vi "Multi_FTP_Put.vi"(0 "Address":string, 1 "User":string, 3 "Password":string, 5 "trj file path 2":path[](array[path]), 7 "Local Files To Put (DOS Wildcards allowed)":string, 9 "XPS error in(no error)":errorcluster, 11 "error in (no error)":errorcluster, 12 "Cible Directory":string) -> (10 "XPS error out":errorcluster, 15 "error out":errorcluster)   [LabVIEW 2009]
panel:
  out "concatenated string 2":string
  out "array":string[][](array[string])
  out "size(s) 2":i32[](array[numeric])
  out "standard output":string
  out "concatenated string":string
  out "String":string
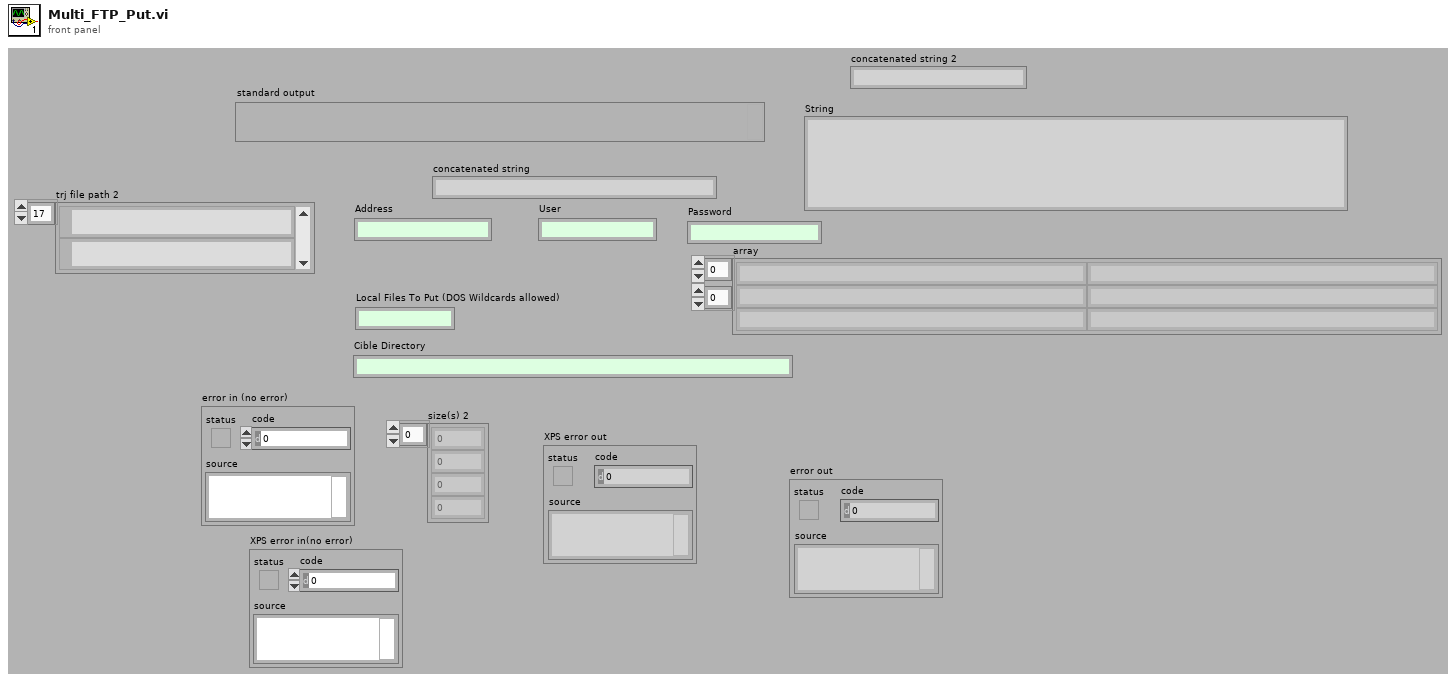
[diagram p1: front panel]
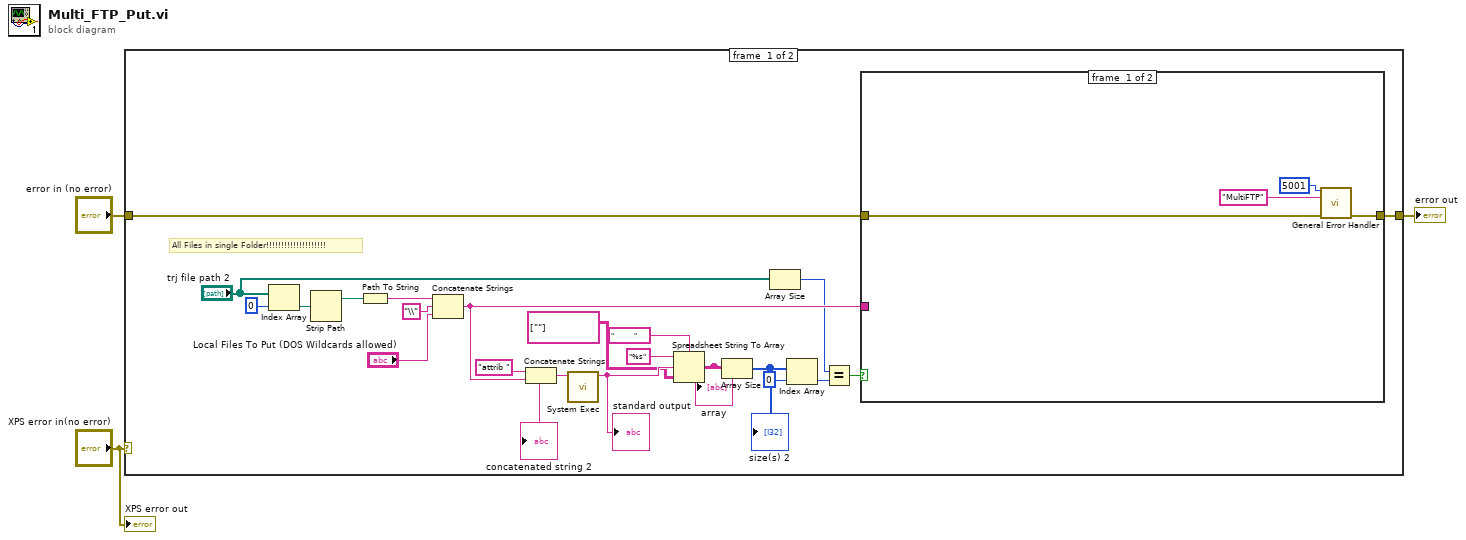
[diagram p0: block diagram]
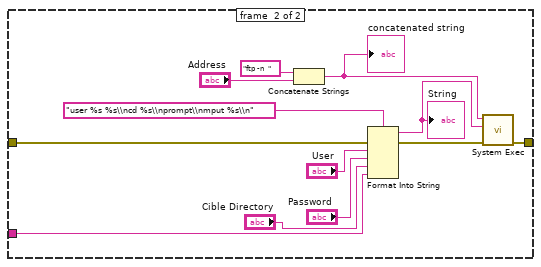
[diagram p2: hidden frame]
diagram:
  n1 = case shown="No Error" "XPS error in(no error)" {
    tunnel: [w25 w42] -> w2
    tunnel: "error in (no error)" -> [w21 w42]
    frame #0 {
      # "All Files in single Folder!!!!!!!!!!!!!!!!!!!!"
      n2 = Index Array(array="trj file path 2", index=0) -> (element=w12:path)
      n3 = Strip Path(path=w12) -> (stripped path=w11:path)  [unwired: 1 out]
      n4 = Path To String(path=w11) -> (string=w23:string)
      n5 = Concatenate Strings(w23, "\\", "Local Files To Put (DOS Wildcards allowed)") -> (w18:string)
      n6 = Concatenate Strings("attrib " ("command line"), w18) -> (w19:string)
      "concatenated string 2" <- w19
      n7 = call <vilib>:"System Exec.vi"("command line"=w19) -> ("standard output"=w17:string)  [unwired: 5 in, 5 out]
      "standard output" <- w17
      n8 = Spreadsheet String To Array(delimiter (Tab)="          ", format string="%s", spreadsheet string=w17, array type (2D Dbl)=string[][] [[""]]) -> (array=w9:string[][])
      "array" <- w9
      n9 = Array Size(array=w9) -> (size(s)=w7:i32[])
      "size(s) 2" <- w7
      n10 = Array Size(array="trj file path 2") -> (size(s)=w4:i32)
      n11 = Index Array(array=w7, index=0) -> (element=w5:i32)
      n12 = Equal?(x=w4, y=w5) -> (x = y?=w8:bool)
      n13 = case shown="True" w8 {
        tunnel: [w28 w34] -> w25
        tunnel: w21 -> [w29 w32]
        tunnel: w18 -> [_ w30]
        frame #0 {
          n14 = call <vilib>:"General Error Handler.vi"("[error code] (0)"=5001, "[error source] (\" \")"="MultiFTP" ("[error source] (\" \")"), "error in (no error)"=w29) -> ("error out"=w28:errorcluster)  [unwired: 8 in, 4 out]
        }
        frame #1 {
          n15 = Concatenate Strings("ftp -n  ", "Address") -> (w39:string)
          "concatenated string" <- w39
          n16 = Format Into String(format string="user %s %s\\ncd %s\\nprompt\\nmput %s\\n", error in=w32, "User", "Password", "Cible Directory", w30) -> (resulting string=w36:string, error out=w35:errorcluster)  [unwired: 1 in]
          "String" <- w36
          n17 = call <vilib>:"System Exec.vi"("error in (no error)"=w35, "standard input"=w36, "command line"=w39) -> ("error out"=w34:errorcluster)  [unwired: 3 in, 5 out]
        }
      }
    }
    frame #1 {
    }
  }
  "error out" <- w2
  "XPS error out" <- "XPS error in(no error)"
